vi "GetHardwareVersion.vi"(8 "error in (no error)":errorcluster caption="Fehler (Eingang, kein Fehler)", 11 "device":u32) -> (0 "error out":errorcluster caption="Fehler (Ausgang)", 2 "function return":u32(ring), 3 "buffer":string)   [LabVIEW 2015, in "IRB.lvlib"]
doc: "irb_result IRB_EXPORT irb_get_hardware_version(irb_device* device, char buffer[]);"
uses:
  IRB.lvlib
  IRB.dll
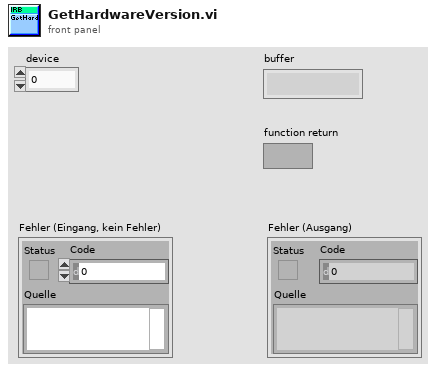
[diagram p1: front panel]
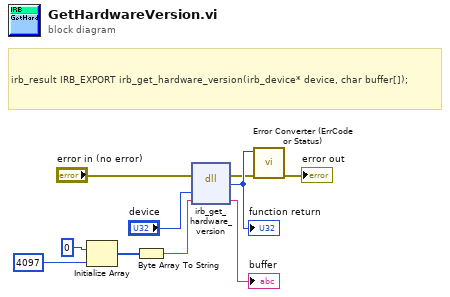
[diagram p0: block diagram]
diagram:
  # "irb_result IRB_EXPORT irb_get_hardware_version(irb_device* device, char buffer[]);"
  n1 = Initialize Array(u8 0 ("Element"), 4097 ("Dimension")) -> (w8:u8[])
  n2 = Byte Array To String(unsigned byte array=w8) -> (string=w7:string)
  n3 = dll-call lib="C:/LabView/IRB/x86_32/IRB.*" fn="irb_get_hardware_version"(error in="error in (no error)", "device"="device", "buffer"=w7) -> (error out=w2:errorcluster, w10:u32, "buffer"=→"buffer":string)  [unwired: 3 in, 1 out]
  "function return" <- w10
  n4 = call "Error Converter (ErrCode or Status).vi"("error in (no error)"=w2, "error code"=w10) -> ("error out"=→"error out":errorcluster)  [unwired: 9 in]
